vi "PCRE Test.vi"(10 "Values Table":string="{\n \"{test}\": 1\n}", 11 "Expression In":string="({test} == true) OR {b} == false AND {c} == ON") -> (0 "error out":errorcluster, 1 "Reverse Polish Notation Token Stack":cluster{string, string}[](array[cluster]), 2 "Tokens":cluster{string, string}[](array[cluster]), 4 "Total Time":dbl format="%.6fsec", 5 "Result":T1, 6 "Compile Time":dbl format="%.6fsec")   [LabVIEW 2014]
uses:
  src/core/expression/FTW-Expr-BooleanExpressionResult.ctl
  src/core/error/FTW-ERR-ThrowError.vi
  src/core/error/FTW-ERR-CallChain.vi
  src/core/string/FTW-STR-ReplaceWhitespace.vi
  src/core/expression/pcre-8.35/builds/Debug/pcred.dll
  lib/pcre/FTWLib-PCRE32.dll
panel:
  out "Match End":i32
  out "Match Begin":i32
  out "ALL Tokens":cluster{string, string}[](array[cluster])
  out "data string":string
  out "error out 3":errorcluster
  out "LabVIEW PCRE":dbl format="%.4psec"
  out "error out 2":errorcluster
  out "Array":string[](array[string])
  out "Subject":string
  out "Callout Data":T2(array[cluster]) {"callout_id" format="%.0x"; "subject_current_pos" format="%.0x"; "subject_start_match_pos" format="%.0x"; "cap_top" format="%.0x"; "cap_last" format="%.0x"; "patt_pos" format="%.0x"}
  out "Submatches":cluster{i32, i32}[](array[cluster])
  out "PCRE Exec Return":i64
  in  "exec starting offset":i32
  out "Error Offset in Pattern":i64
  out "Error String":string
  out "Pattern":string
  # "({test} == true) OR {b} == false AND {c} == ON"
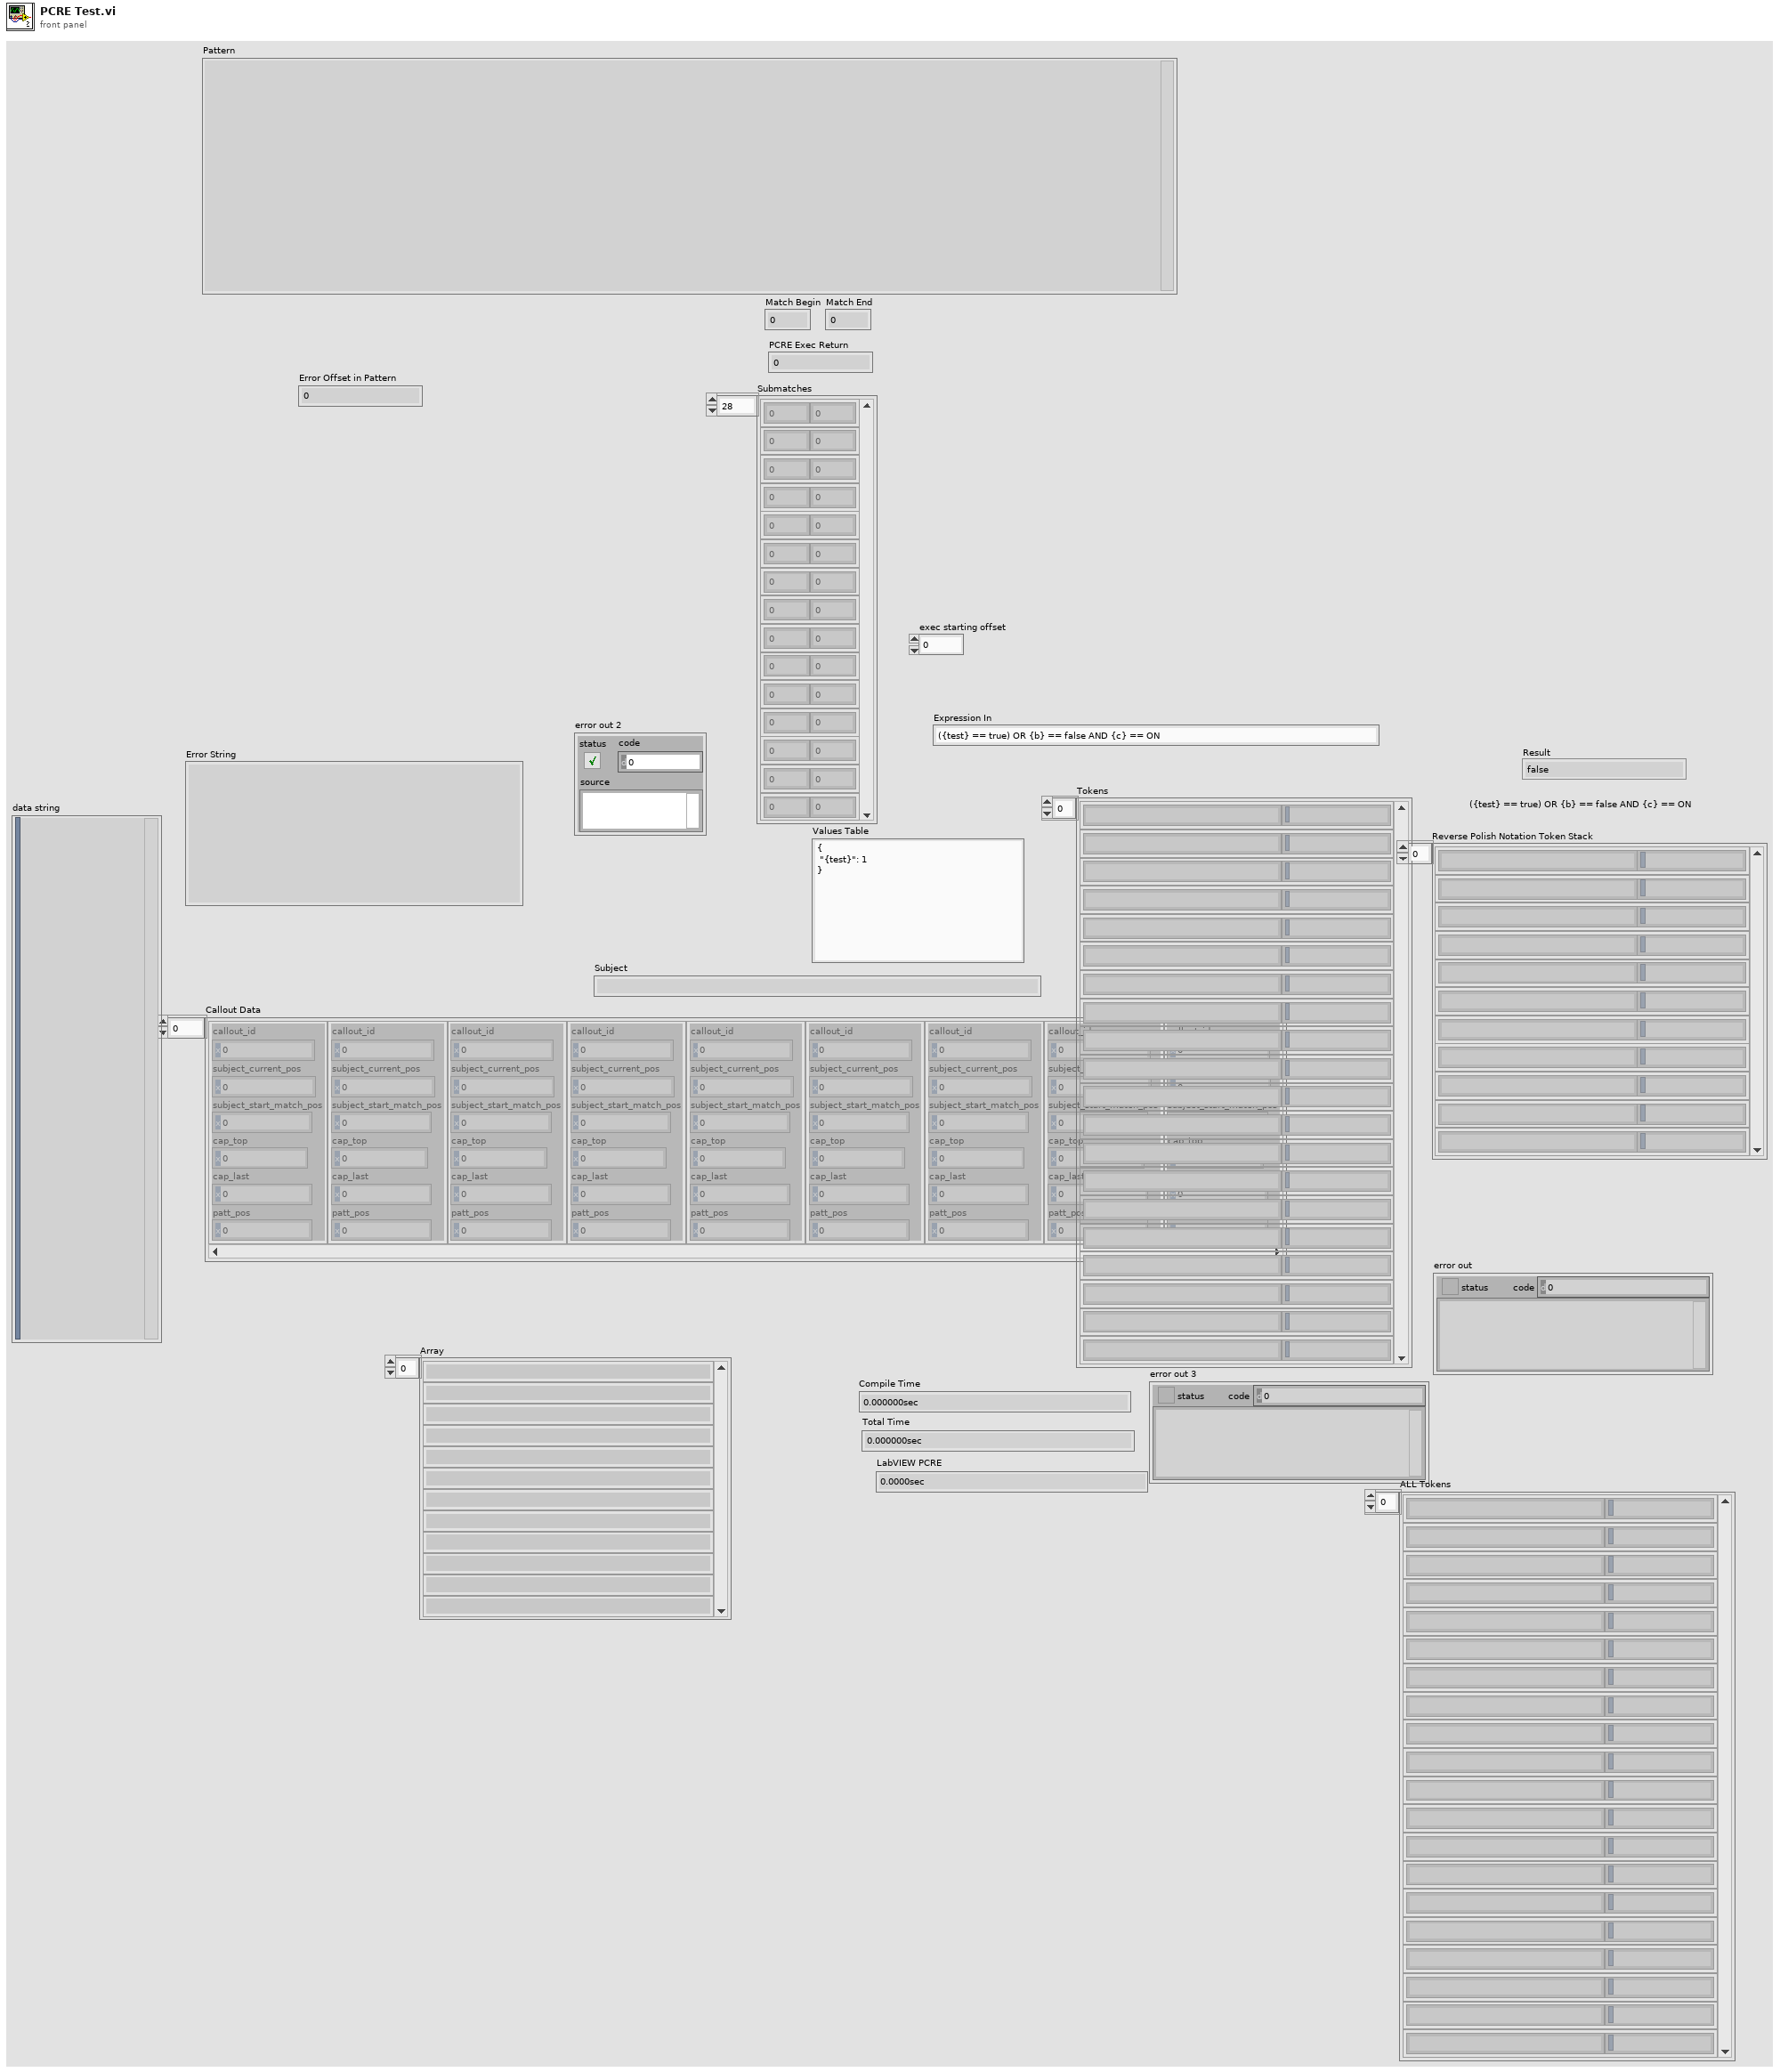
[diagram p1: front panel]
types:
  T1 = typedef "FTW-Expr-BooleanExpressionResult.ctl" = enum16{"false", "true", "inconclusive"}
  T2 = cluster{"callout_id":i32, "subject_current_pos":i32, "subject_start_match_pos":i32, "cap_top":i32, "cap_last":i32, "patt_pos":i32}[]
  T3 = cluster{"op":cluster{"token":string, "value":string}, "Precedence":i32, "Scope Depth":i32}[]
  T4 = cluster{"callout_id":i32, "subject_current_pos":i32, "subject_start_match_pos":i32, "cap_top":i32, "cap_last":i32, "patt_pos":i32}
  T5 = cluster{cluster{"token":string, "value":string}, "Precedence":i32, i32}
  T6 = cluster{"op":cluster{"token":string, "value":string}, "Precedence":i32, "Scope Depth":i32}
  T7 = cluster{cluster{"token":string, "value":string}, "default value 1":i32, "Current Scope Depth":i32}
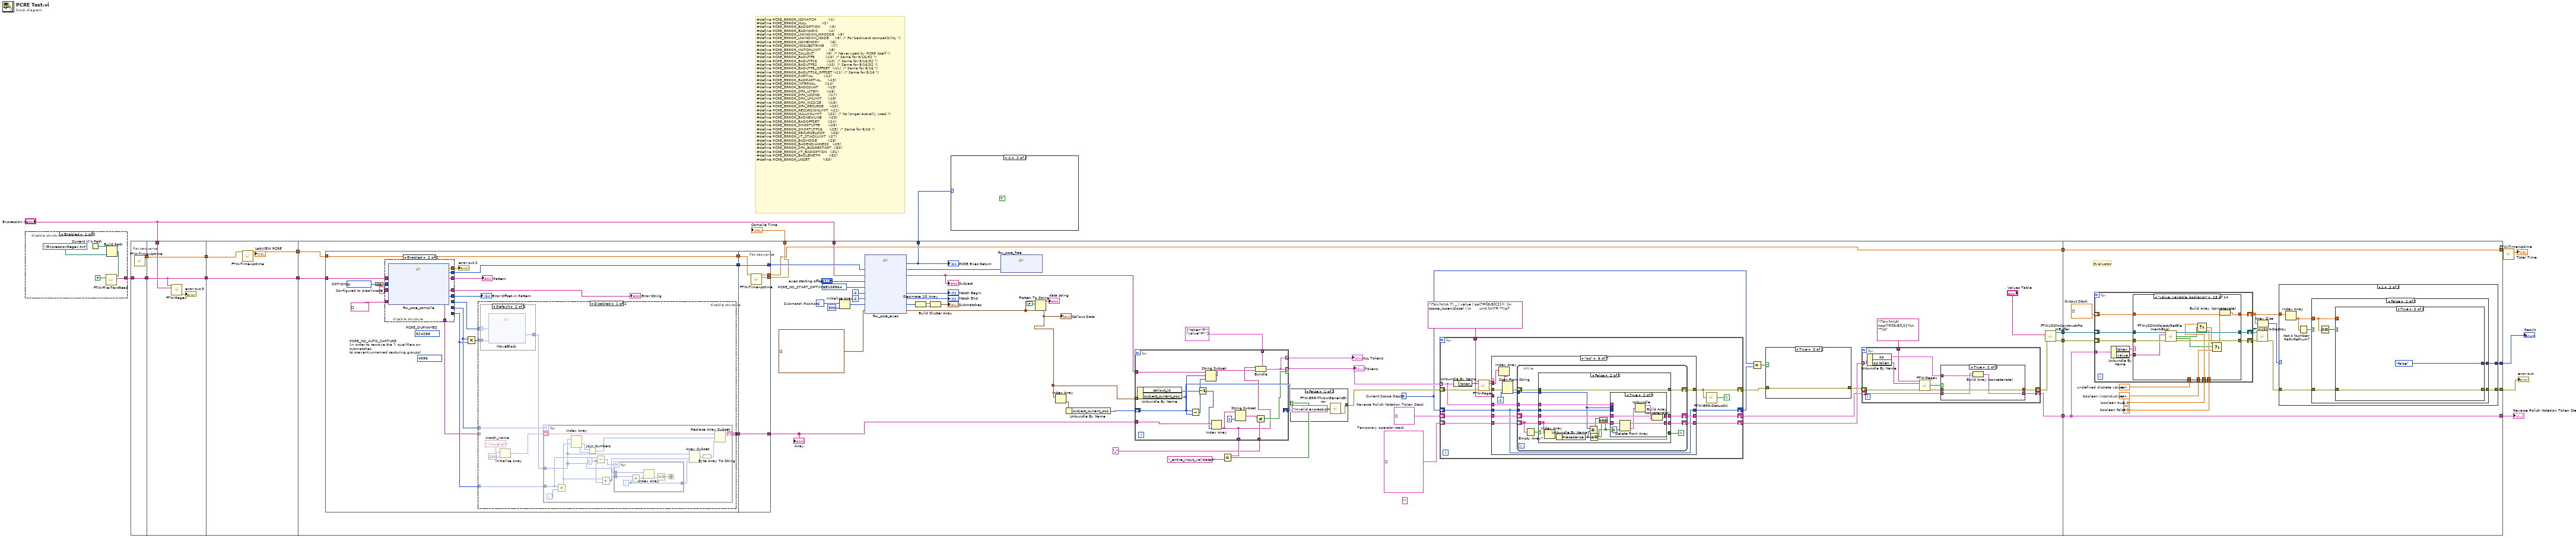
[diagram p0: block diagram]
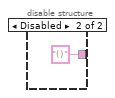
[diagram p3: hidden frame]
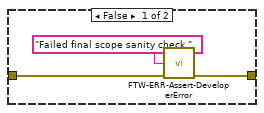
[diagram p4: hidden frame]
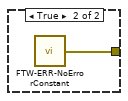
[diagram p5: hidden frame]
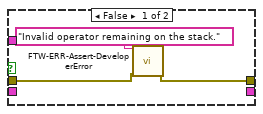
[diagram p6: hidden frame]
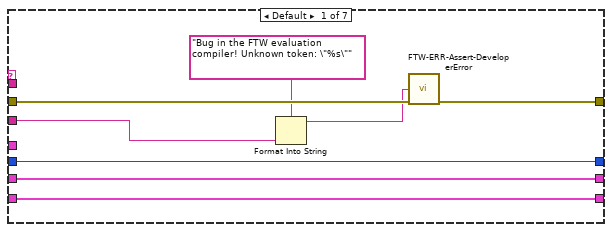
[diagram p7: hidden frame]
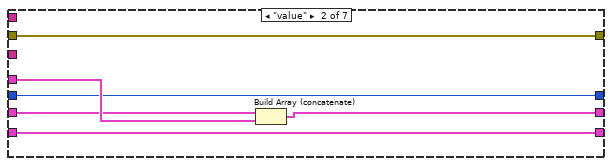
[diagram p8: hidden frame]
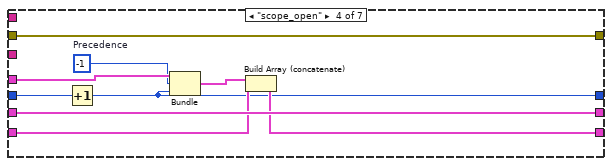
[diagram p10: hidden frame]
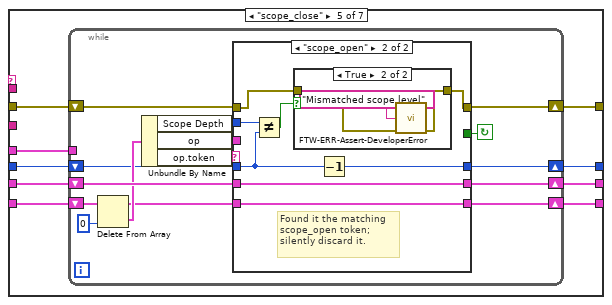
[diagram p11: hidden frame]
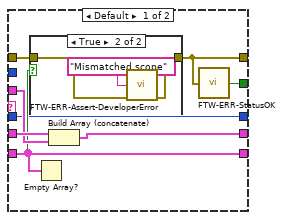
[diagram p12: hidden frame]
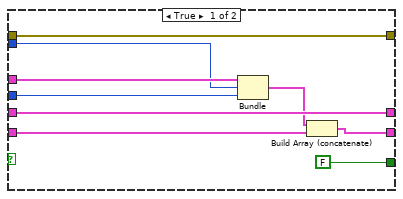
[diagram p15: hidden frame]
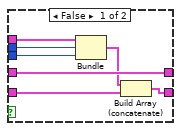
[diagram p16: hidden frame]
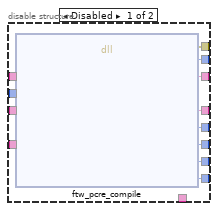
[diagram p20: hidden frame]
diagram:
  # "#define PCRE_ERROR_NOMATCH          (-1)\n#define PCRE_ERROR_NULL             (-2)\n#define PCRE_ERROR_BADOPTION        (-3)\n#define PCRE_ERROR_BADMAGIC         (-4)\n#define PCRE_ERROR_UNKNOWN_OPCODE   (-5)\n#define PCRE_ERROR_UNKNOWN_NODE     (-5)  /* For backward compatibility */\n#define PCRE_ERROR_NOMEMORY         (-6)\n#define PCRE_ERROR_NOSUBSTRING      (-7)\n#define PCRE_ERROR_MATCHLIMIT       (-8)\n#define PCRE_ERROR_CALLOUT          (-9)  /* Never used by PCRE itself */\n#define PCRE_ERROR_BADUTF8         (-10)  /* Same for 8/16/32 */\n#define PCRE_ERROR_BADUTF16        (-10)  /* Same for 8/16/32 */\n#define PCRE_ERROR_BADUTF32        (-10)  /* Same for 8/16/32 */\n#define PCRE_ERROR_BADUTF8_OFFSET  (-11)  /* Same for 8/16 */\n#define PCRE_ERROR_BADUTF16_OFFSET (-11)  /* Same for 8/16 */\n#define PCRE_ERROR_PARTIAL         (-12)\n#define PCRE_ERROR_BADPARTIAL      (-13)\n#define PCRE_ERROR_INTERNAL        (-14)\n#define PCRE_ERROR_BADCOUNT        (-15)\n#define PCRE_ERROR_DFA_UITEM       (-16)\n#define PCRE_ERROR_DFA_UCOND       (-17)\n#define PCRE_ERROR_DFA_UMLIMIT     (-18)\n#define PCRE_ERROR_DFA_WSSIZE      (-19)\n#define PCRE_ERROR_DFA_RECURSE     (-20)\n#define PCRE_ERROR_RECURSIONLIMIT  (-21)\n#define PCRE_ERROR_NULLWSLIMIT     (-22)  /* No longer actually used */\n#define PCRE_ERROR_BADNEWLINE      (-23)\n#define PCRE_ERROR_BADOFFSET       (-24)\n#define PCRE_ERROR_SHORTUTF8       (-25)\n#define PCRE_ERROR_SHORTUTF16      (-25)  /* Same for 8/16 */\n#define PCRE_ERROR_RECURSELOOP     (-26)\n#define PCRE_ERROR_JIT_STACKLIMIT  (-27)\n#define PCRE_ERROR_BADMODE         (-28)\n#define PCRE_ERROR_BADENDIANNESS   (-29)\n#define PCRE_ERROR_DFA_BADRESTART  (-30)\n#define PCRE_ERROR_JIT_BADOPTION   (-31)\n#define PCRE_ERROR_BADLENGTH       (-32)\n#define PCRE_ERROR_UNSET           (-33)"
  n1 = disable-structure shown="Enabled" {
    disable-tunnel: [w21 "()" ("Text")] -> w19
    frame Enabled {
      n2 = Current VI's Path() -> (path=w22:path)
      n3 = Build Path(base path=w22, name or relative path=path "../ExpressionRegex.txt" ("path")) -> (appended path=w20:path)
      n4 = call "FTW-File-TextRead.vi"("Filepath"=w20, "Create if doesn't exist?"=FALSE) -> ("Text"=w21:string)  [unwired: 11 in, 2 out]
    }
    frame Disabled {
    }
  }
  n5 = flat-sequence {
    tunnel: w19 -> [w27]
    tunnel: [w27] -> w6
    tunnel: [w26] -> w2
    tunnel: w6 -> [w31]
    tunnel: [w31] -> w5
    tunnel: "Expression In" -> [w30]
    tunnel: [w29] -> w3
    tunnel: w2 -> [w29]
    tunnel: [w34] -> w16
    tunnel: [w35] -> w14
    tunnel: w5 -> [w34]
    tunnel: w3 -> [w33]
    tunnel: "Expression In" -> [w78]
    tunnel: w16 -> [w83]
    tunnel: w14 -> [w66]
    tunnel: [w61] -> w12
    tunnel: [w57] -> w11
    tunnel: [w67] -> w10
    tunnel: [w62] -> w9
    tunnel: [w60] -> w8
    tunnel: [w36] -> w1
    tunnel: [w379] -> w15
    tunnel: [w378] -> w17
    tunnel: [w370] -> w18
    tunnel: w11 -> [w375]
    tunnel: w10 -> [w378]
    tunnel: w9 -> [w379]
    tunnel: w8 -> [w376]
    tunnel: [w365] -> w7
    frame #0 {
      n6 = call "FTW-Time-Uptime.vi"() -> ("Current Uptime"=w26:dbl)  [unwired: 13 in, 2 out]
    }
    frame #1 {
      n7 = call "FTW-Regex.vi"("Regular Expression"=w31, "Input String"=w30) -> ("error out"=→"error out 3":errorcluster)  [unwired: 9 in, 4 out]
    }
    frame #2 {
      n8 = call "FTW-Time-Uptime.vi"("Previous Uptime"=w33) -> ("Current Uptime"=w35:dbl, "Elapsed Time"=→"LabVIEW PCRE":dbl)  [unwired: 12 in, 1 out]
    }
    frame #3 {
      w39 = -2  # Submatch Position
      (unwired) ""
      w54 = 0  # Current Scope Depth
      w71 = T3 []  # Temporary operator stack
      w72 = cluster{"token":string, "value":string}[] []  # Reverse Polish Notation Token Stack
      w82 = 67108864  # PCRE_NO_START_OPTIMIZE
      n9 = flat-sequence {
        tunnel: w83 -> [w280]
        tunnel: w66 -> [w276]
        tunnel: [w285] -> w65
        tunnel: [w279] -> w64
        tunnel: [w276] -> w63
        tunnel: [w346] -> w80
        tunnel: [w347] -> w90
        tunnel: w65 -> [w347]
        tunnel: w64 -> [w346]
        tunnel: w63 -> [w343]
        tunnel: [w345] -> w62
        tunnel: [w344] -> w61
        frame #0 {
          w273 = ""  # Configured to preallocate
          (unwired) 4096  # PCRE_NO_AUTO_CAPTURE (in order to remove the ?: qualifiers on submatches to prevent unnamed capturing groups)
          (unwired) 524288  # PCRE_DUPNAMES
          w278 = 0  # OPTIONS
          n10 = Compound Arithmetic op=OR(w278) -> (w277:i32)
          n11 = disable-structure shown="Enabled" {
            disable-tunnel: [w332 w342] -> w287
            disable-tunnel: [w331 w341] -> w286
            disable-tunnel: [w330 w340] -> w285
            disable-tunnel: [w329 _] -> w284
            disable-tunnel: [w328 _] -> w282
            disable-tunnel: [w327 _] -> w281
            disable-tunnel: w280 -> [w326 w339]
            disable-tunnel: w277 -> [w325 w338]
            disable-tunnel: [w324 w337] -> w275
            disable-tunnel: [w323 w336] -> w274
            disable-tunnel: w273 -> [w322 w335]
            disable-tunnel: string[] [] ("initialized array") -> [_ w334]
            disable-tunnel: [_ w333] -> w271
            frame Disabled {
              n12 = dll-call lib="C:/Users/Jack/Desktop/app/Sandbox/Expression Lexer/pcre-8.35/builds/Debug/pcred.dll" fn="ftw_pcre_compile"("Pattern"=w326, "Options"=w325, "Error String"=w322) -> (error out=w324:errorcluster, "Compiled Regex"=w330:i64, "Pattern"=w332:string, "Error String"=w323:string, "Error Offset in Pattern"=w331:i64, "Named Capturing Group Table*"=w329:i64, "Named Capturing Group Count"=w328:i32, "Named Capturing Group Length"=w327:i32)  [unwired: 8 in, 1 out]
            }
            frame Enabled {
              n13 = dll-call lib="C:/Users/Jack/repo/ftw-master/ftw/lib/pcre/FTWLib-PCRE32.dll" fn="ftw_pcre_compile"("Pattern"=w339, "Options"=w338, "Error String"=w335, "Named Capturing Group Table"=w334) -> (error out=w337:errorcluster, "Compiled Regex"=w340:i64, "Pattern"=w342:string, "Error String"=w336:string, "Error Offset in Pattern"=w341:i64, "Named Capturing Group Table"=w333:string[])  [unwired: 5 in, 1 out]
            }
          }
          "Pattern" <- w287
          "Error String" <- w274
          "Error Offset in Pattern" <- w286
          "error out 2" <- w275
          n14 = Multiply(x=w282, y=w281) -> (x*y=w283:i32)
          n15 = disable-structure shown="Disabled" {
            disable-tunnel: w284 -> [w296 _]
            disable-tunnel: w283 -> [w295 _]
            disable-tunnel: w282 -> [w294 _]
            disable-tunnel: w281 -> [w293 _]
            disable-tunnel: [w288 w321] -> w279
            disable-tunnel: w271 -> [_ w321]
            frame Disabled {
              w289 = "<invalid>"  # match_name
              n16 = case shown="Default" w296 {
                selector: w296 -> [_ w319]
                tunnel: [_ w320] -> w292
                tunnel: w295 -> [_ w318]
                frame 0 {
                }
                frame Default {
                  n17 = dll-call lib="LabVIEW" fn="MoveBlock"("Source Pointer"=w319, "Buffer Size"=w318) -> ("Destination Buffer"=w320:u8[])  [unwired: 7 in, 2 out]
                }
              }
              n18 = Initialize Array(w289, 256 ("dimension size")) -> (w290:string[])
              n19 = for {
                N: w294 -> [_]
                tunnel: w293 -> [w308]
                tunnel: w292 -> [w304]
                shift-right: [w297] -> w288
                shift-left: w290 -> [w300]
                i -> [w311]
                w306 = 2 ("y")
                n20 = Multiply(x=w308, y=w311) -> (x*y=w305:i32)
                n21 = Index Array(array=w304, index #1=w305) -> (element #1=w310:u8, element #2=w309:u8)  [unwired: 1 in]
                n22 = Join Numbers(hi=w310, lo=w309) -> ((hi.lo)=w299:u16)
                n23 = Subtract(x=w308, y=w306) -> (x-y=w307:i32)
                n24 = Add(x=w305, y=w306) -> (x+y=w301:i32)
                n25 = for {
                  N: w307 -> [_]
                  tunnel: w304 -> [w317]
                  tunnel: w301 -> [w316]
                  tunnel: [w312] -> w302
                  i -> [w312]
                  stop <- w313 stop-if-true
                  n26 = Add(x=w316, y=w312) -> (x+y=w315:i32)
                  n27 = Index Array(array=w317, index=w315) -> (element=w314:u8)
                  n28 = Equal To 0?(x=w314) -> (x = 0?=w313:bool)
                }
                n29 = Array Subset(array=w304, index=w301, length=w302) -> (w303:u8[])
                n30 = Byte Array To String(unsigned byte array=w303) -> (string=w298:string)
                n31 = Replace Array Subset(array=w300, new element=w298, index=w299) -> (w297:string[])
              }
            }
            frame Enabled {
            }
          }
        }
        frame #1 {
          n32 = call "FTW-Time-Uptime.vi"("Previous Uptime"=w343) -> ("Current Uptime"=w345:dbl, "Elapsed Time"=w344:dbl)  [unwired: 12 in, 1 out]
        }
      }
      n33 = Initialize Array(w39, 300 ("dimension size")) -> (w37:i32[])
      n34 = dll-call lib="C:/Users/Jack/repo/ftw-master/ftw/lib/pcre/FTWLib-PCRE32.dll" fn="ftw_pcre_exec"("Compiled Expression"=w90, "Subject String"=w78, "Starting Offset"="exec starting offset", "Options"=w82, "Match Begin"=-2, "Match End"=-2, "Submatch Buffer"=w37, "Callout Buffer"=T2 [] ("*(type *) &x")) -> ("Return Value"=w36:i64, "Compiled Expression"=w49:i64, "Subject String"=w81:string, "Match Begin"=→"Match Begin":i32, "Match End"=→"Match End":i32, "Submatch Buffer"=w89:i32[], "Callout Buffer"=w47:T2)  [unwired: 5 in, 2 out]
      "PCRE Exec Return" <- w36
      "Callout Data" <- w47
      "Subject" <- w81
      n35 = Decimate 1D Array(w89) -> (w88:i32[], w87:i32[])
      n36 = Build Cluster Array(w88, w87) -> (→"Submatches":cluster{i32, i32}[])
      n37 = dll-call lib="C:/Users/Jack/repo/ftw-master/ftw/lib/pcre/FTWLib-PCRE32.dll" fn="ftw_pcre_free"("Compiled Expression"=w49) -> ()  [unwired: 5 in, 2 out]
      n38 = Flatten To String(anything=w47, prepend array or string size? (T)=FALSE) -> (data string=→"data string":string)  [unwired: 2 in, 2 out]
      n39 = Index Array(array=w47) -> (element=w85:T4)  [unwired: 1 in]
      n40 = Unbundle By Name(w85) -> ("subject_current_pos"=w84:i32)
      n41 = for {
        tunnel: w47 -> [w363] mode=indexing
        shift-right: [w360] -> _
        shift-left: w84 -> [w361]
        tunnel: w81 -> [w359]
        tunnel: [w348] -> w75 mode=indexing if=w354
        tunnel: w80 -> [w358]
        tunnel: [w352] -> w77
        tunnel: "_" -> [w356]
        tunnel: cluster{"token":string, "value":string} {"token"="", "value"=""} -> [w353]
        tunnel: [w348] -> w44 mode=indexing
        n42 = Unbundle By Name(w363) -> ("callout_id"=w350:i32, "subject_current_pos"=w360:i32)
        n43 = Subtract(x=w360, y=w361) -> (x-y=w362:i32)
        n44 = Decrement(x=w350) -> (x-1=w349:i32)
        n45 = String Subset(string=w359, offset (0)=w361, length (rest)=w362) -> (substring=w351:string)
        n46 = Index Array(array=w358, index=w349) -> (element=w352:string)
        n47 = String Subset(string=w352, length (rest)=1 ("length (rest)")) -> (substring=w357:string)  [unwired: 1 in]
        n48 = Not Equal?(x=w357, y=w356) -> (x != y?=w354:bool)
        n49 = Bundle(cluster=w353, "token"=w352, "value"=w351) -> (w348:cluster{"token":string, "value":string})
      }
      "Tokens" <- w75
      "ALL Tokens" <- w44
      n50 = Equal?(x=w77, y="_entire_input_validated") -> (x = y?=w56:bool)
      n51 = case shown="False" w56 {
        tunnel: [w96 w98] -> w55
        frame False {
          n52 = call "FTW-ERR-ThrowGenericError.vi"("Error Message"="Invalid expression") -> ("error out"=w96:errorcluster)  [unwired: 14 in]
        }
        frame True {
          n53 = call "FTW-ERR-NoErrorConstant.vi"() -> ("no error"=w98:errorcluster)
        }
      }
      n54 = for {
        tunnel: w75 -> [w127] mode=indexing
        tunnel: "(?six)\n\\A (?: _ | value | op(?=([0-9]{2}))  |\n       scope_(open|close) | \n       unit )\n(?=.*?\\z)" ("Regular Expression") -> [w130]
        shift-right: [w125] -> w68
        shift-left: w72 -> [w126]
        shift-right: [w122] -> w51
        shift-left: w55 -> [w124]
        shift-right: [w120] -> w70
        shift-left: w71 -> [w119]
        shift-right: [w116] -> w53
        shift-left: w54 -> [w117]
        stop <- w121 continue-if-true
        n55 = Unbundle By Name(w127) -> ("token"=w118:string)
        n56 = call "FTW-Regex.vi"("Regular Expression"=w130, "Input String"=w118, "error in"=w124) -> ("Match"=w129:string, "Submatches"=w128:string[], "error out"=w123:errorcluster)  [unwired: 8 in, 2 out]
        n57 = case shown="\"op\"" w129 {
          tunnel: w128 -> [_ _ _ _ _ w209 _]
          tunnel: w127 -> [_ w144 _ w153 w162 w210 _]
          tunnel: w126 -> [w136 w143 w147 w156 w166 w214 w269]
          tunnel: [w136 w142 w147 w156 w164 w215 w269] -> w125
          tunnel: [w137 w141 w148 w157 w161 w212 w270] -> w122
          tunnel: w123 -> [w138 w141 w148 w157 w160 w219 w270]
          tunnel: [w135 w140 w146 w154 w163 w211 w268] -> w120
          tunnel: w119 -> [w135 w140 w146 w155 w165 w216 w268]
          tunnel: w118 -> [w132 _ _ _ _ _ _]
          tunnel: w117 -> [w131 w139 w145 w151 w159 w207 w267]
          tunnel: [w131 w139 w145 w150 w158 w207 w267] -> w116
          frame Default {
            n58 = Format Into String(format string="Bug in the FTW evaluation compiler! Unknown token: \"%s\"" ("Reason this error should never happen"), w132) -> (resulting string=w133:string)  [unwired: 2 in, 1 out]
            n59 = call "FTW-ERR-Assert-DeveloperError.vi"("Reason this error should never happen"=w133, "error in"=w138) -> ("error out"=w137:errorcluster)  [unwired: 13 in]
          }
          frame "value" {
            n60 = Build Array (concatenate)(w143, w144) -> (w142:cluster{"token":string, "value":string}[])
          }
          frame "_" {
            # "As a convention, ignore tokens\nthat begin with this character.\nThey exist in the callout array in\norder to maintain match position."
          }
          frame "scope_open" {
            w149 = -1  # Precedence
            n61 = Increment(x=w151) -> (x+1=w150:i32)
            n62 = Bundle(w153, "Precedence"=w149, w150) -> (w152:T5)  [unwired: 1 in]
            n63 = Build Array (concatenate)(w152, w155) -> (w154:T3)
          }
          frame "scope_close" {
            n64 = while {
              shift-right: [w172] -> w161
              shift-left: w160 -> [w173]
              shift-right: [w181] -> w164
              shift-left: w166 -> [w180]
              shift-right: [w179] -> w163
              shift-left: w165 -> [w178]
              tunnel: w162 -> [_]
              shift-right: [w169] -> w158
              shift-left: w159 -> [w168]
              stop <- w170 continue-if-true
              n65 = Delete From Array(array=w178, index=0) -> (deleted portion=w176:T6, array with subset deleted=w174:T3)  [unwired: 1 in]
              n66 = Unbundle By Name(w176) -> ("Scope Depth"=w167:i32, "op"=w171:cluster{"token":string, "value":string}, "op.token"=w175:string)
              n67 = case shown="\"scope_open\"" w175 {
                tunnel: [w190 w202] -> w181
                tunnel: w180 -> [w189 w202]
                tunnel: [w186 w201] -> w179
                tunnel: w174 -> [w186 w201]
                tunnel: w173 -> [w187 w197]
                tunnel: [w184 w196] -> w172
                tunnel: w171 -> [w188 _]
                tunnel: [w183 _] -> w170
                tunnel: [w182 w200] -> w169
                tunnel: w168 -> [w182 w198]
                tunnel: w167 -> [_ w199]
                frame Default {
                  n68 = Empty Array?(array=w186) -> (empty?=w185:bool)
                  n69 = case shown="True" w185 {
                    tunnel: w187 -> [w191 w194]
                    tunnel: [w191 w192] -> w184
                    frame False {
                    }
                    frame True {
                      n70 = call "FTW-ERR-Assert-DeveloperError.vi"("Reason this error should never happen"="Mismatched scope", "error in"=w194) -> ("error out"=w192:errorcluster)  [unwired: 13 in]
                    }
                  }
                  n71 = Build Array (concatenate)(w189, w188) -> (w190:cluster{"token":string, "value":string}[])
                  n72 = call "FTW-ERR-StatusOK.vi"("error to check"=w184) -> ("Status OK?"=w183:bool)
                }
                frame "scope_open" {
                  # "Found it the matching\nscope_open token;\nsilently discard it."
                  n73 = Not Equal?(x=w199, y=w198) -> (x != y?=w195:bool)
                  n74 = case shown="True" w195 {
                    tunnel: w197 -> [w203 w206]
                    tunnel: [w203 w204] -> w196
                    frame False {
                    }
                    frame True {
                      n75 = call "FTW-ERR-Assert-DeveloperError.vi"("Reason this error should never happen"="Mismatched scope level", "error in"=w206) -> ("error out"=w204:errorcluster)  [unwired: 13 in]
                    }
                  }
                  n76 = Decrement(x=w198) -> (x-1=w200:i32)
                }
              }
            }
          }
          frame "op" {
            n77 = Index Array(array=w209) -> (element=w208:string)  [unwired: 1 in]
            n78 = Scan From String(input string=w208, error in=w219, default 1=-1 ("default value 1")) -> (error out=w213:errorcluster, output 1=w217:i32)  [unwired: 2 in, 2 out]
            n79 = while {
              tunnel: w217 -> [w225]
              shift-right: [w221] -> w212
              shift-left: w213 -> [w220]
              shift-right: [w230] -> w215
              shift-left: w214 -> [w229]
              shift-right: [w228] -> w211
              shift-left: w216 -> [w227]
              tunnel: w210 -> [w226]
              tunnel: w207 -> [w224]
              stop <- w222 continue-if-true
              n80 = Empty Array?(array=w227) -> (empty?=w223:bool)
              n81 = case shown="False" w223 {
                tunnel: [w239 w252] -> w230
                tunnel: w229 -> [w239 w251]
                tunnel: [w238 w250] -> w228
                tunnel: w227 -> [w237 w246]
                tunnel: w226 -> [w236 w249]
                tunnel: w225 -> [w235 w248]
                tunnel: w224 -> [w234 w247]
                tunnel: [FALSE w240] -> w222
                tunnel: [w231 w244] -> w221
                tunnel: w220 -> [w231 w244]
                frame True {
                  n82 = Bundle(w236, "default value 1"=w235, "Current Scope Depth"=w234) -> (w233:T7)  [unwired: 1 in]
                  n83 = Build Array (concatenate)(w233, w237) -> (w238:T3)
                }
                frame False {
                  n84 = Index Array(array=w246) -> (element=w245:T6)  [unwired: 1 in]
                  n85 = Unbundle By Name(w245) -> ("Precedence"=w243:i32)
                  n86 = Greater Or Equal?(x=w248, y=w243) -> (x >= y?=w242:bool)
                  n87 = Greater Or Equal To 0?(x=w243) -> (x >= 0?=w241:bool)
                  n88 = And(x=w242, y=w241) -> (x .and. y?=w240:bool)
                  n89 = case shown="True" w240 {
                    tunnel: [w259 w265] -> w252
                    tunnel: w251 -> [w259 w266]
                    tunnel: [w257 w260] -> w250
                    tunnel: w246 -> [w258 w261]
                    tunnel: w249 -> [w256 _]
                    tunnel: w248 -> [w255 _]
                    tunnel: w247 -> [w253 _]
                    frame False {
                      n90 = Bundle(w256, "default value 1"=w255, "Current Scope Depth"=w253) -> (w254:T7)  [unwired: 1 in]
                      n91 = Build Array (concatenate)(w254, w258) -> (w257:T3)
                    }
                    frame True {
                      n92 = Delete From Array(array=w261, index=0) -> (deleted portion=w263:T6, array with subset deleted=w260:T3)  [unwired: 1 in]
                      n93 = Unbundle(w263) -> ("op"=w262:cluster{"token":string, "value":string})  [unwired: 2 out]
                      n94 = Build Array (concatenate)(w266, w262) -> (w265:cluster{"token":string, "value":string}[])
                    }
                  }
                }
              }
            }
          }
          frame "unit" {
          }
        }
        n95 = call "FTW-ERR-StatusOK.vi"("error to check"=w122) -> ("Status OK?"=w121:bool)
      }
      n96 = Equal?(x=w54, y=w53) -> (x = y?=w52:bool)
      n97 = case shown="True" w52 {
        tunnel: w51 -> [w93 w95]
        tunnel: [w92 w95] -> w50
        frame False {
          n98 = call "FTW-ERR-Assert-DeveloperError.vi"("Reason this error should never happen"="Failed final scope sanity check.", "error in"=w93) -> ("error out"=w92:errorcluster)  [unwired: 13 in]
        }
        frame True {
        }
      }
      n99 = for {
        tunnel: w70 -> [w108] mode=indexing
        shift-right: [w102] -> w58
        shift-left: w50 -> [w107]
        tunnel: "(?six)\n\\A\nop(?=([0-9]{2}))\n.*?\\z" ("Regular Expression") -> [w105]
        shift-right: [w99] -> w67
        shift-left: w68 -> [w100]
        n100 = Unbundle By Name(w108) -> ("op"=w101:cluster{"token":string, "value":string}, "op.token"=w106:string)
        n101 = call "FTW-Regex.vi"("Regular Expression"=w105, "Input String"=w106, "error in"=w107) -> ("Match Found?"=w104:bool, "error out"=w103:errorcluster)  [unwired: 8 in, 3 out]
        n102 = case shown="True" w104 {
          tunnel: w103 -> [w111 w115]
          tunnel: [w109 w115] -> w102
          tunnel: w101 -> [_ w114]
          tunnel: w100 -> [_ w113]
          tunnel: [_ w112] -> w99
          frame False {
            n103 = call "FTW-ERR-Assert-DeveloperError.vi"("Reason this error should never happen"="Invalid operator remaining on the stack.", "error in"=w111) -> ("error out"=w109:errorcluster)  [unwired: 13 in]
          }
          frame True {
            n104 = Build Array (concatenate)(w113, w114) -> (w112:cluster{"token":string, "value":string}[])
          }
        }
      }
      n105 = call "FTW-JSON-Construct-FromBuffer.vi"("JSON String (UTF-8)"="Values Table", "error in"=w58) -> ("JSON Object"=w60:refnum<data-value>, "error out"=w57:errorcluster)  [unwired: 12 in]
      "Array" <- w80
    }
    frame #4 {
      w364 = nan  # undefined discrete value
      w366 = nan  # boolean inconclusive
      w367 = 1.0  # boolean true
      w368 = 0.0  # boolean false
      w377 = dbl[] []  # Output Stack
      # "Evaluator"
      n106 = for {
        tunnel: w378 -> [w423] mode=indexing
        shift-right: [w420] -> w369
        shift-left: w377 -> [w421]
        shift-right: [w418] -> w374
        shift-left: w376 -> [w419]
        shift-right: [w416] -> w373
        shift-left: w375 -> [w417]
        tunnel: w368 -> [w414]
        tunnel: w367 -> [w413]
        tunnel: w366 -> [w412]
        tunnel: w364 -> [w411]
        n107 = Unbundle By Name(w423) -> ("token"=w422:string, "value"=w415:string)
        n108 = case shown="\"value_variable_boolexpr\"" w422 {
          selector: w422 -> [w425 _ _ _ _ _ _ _ _ _ _ _ _ _]
          tunnel: w421 -> [w431 w450 w469 w490 w511 w530 w544 w549 w554 w559 w564 w569 w579 w591]
          tunnel: [w431 w444 w463 w485 w506 w525 w542 w548 w552 w557 w563 w568 w578 w590] -> w420
          tunnel: w419 -> [w430 w443 w462 w484 w505 w524 w541 w547 w551 w556 w562 w567 w583 w595]
          tunnel: [w430 w443 w462 w484 w505 w524 w541 w547 w551 w556 w562 w567 w582 w594] -> w418
          tunnel: w417 -> [w429 w442 w461 w483 w504 w523 w540 w546 w550 w555 w561 w566 w581 w593]
          tunnel: [w428 w442 w461 w483 w504 w523 w540 w546 w550 w555 w561 w566 w580 w592] -> w416
          tunnel: w415 -> [w424 _ _ _ _ _ _ _ _ _ _ _ w577 w589]
          tunnel: w414 -> [_ w434 w453 w477 w498 w517 w533 _ _ _ w560 _ w572 _]
          tunnel: w413 -> [_ w433 w452 w472 w493 w515 w532 w545 _ _ _ _ w573 _]
          tunnel: w412 -> [_ w432 w451 w476 w497 w516 w538 _ _ _ _ w565 w574 _]
          tunnel: w411 -> [_ _ _ _ _ _ _ _ _ _ _ _ _ w587]
          frame Default {
            n109 = Format Into String(format string="Unhandled token '%s' with value '%s'" ("Reason this error should never happen"), w425, w424) -> (resulting string=w427:string)  [unwired: 2 in, 1 out]
            n110 = call "FTW-ERR-Assert-DeveloperError.vi"("Reason this error should never happen"=w427, "error in"=w429) -> ("error out"=w428:errorcluster)  [unwired: 13 in]
          }
          frame "op09_infix_discrete_equal" {
            n111 = Delete From Array(array=w450, index=0) -> (deleted portion=w440:dbl, array with subset deleted=w448:dbl[])  [unwired: 1 in]
            n112 = Delete From Array(array=w448, index=0) -> (deleted portion=w441:dbl, array with subset deleted=w445:dbl[])  [unwired: 1 in]
            n113 = Not A Number/Path/Refnum?(number/path/refnum=w440) -> (NaN/Path/Refnum?=w438:bool)
            n114 = Equal?(x=w441, y=w440) -> (x = y?=w446:bool)
            n115 = Not A Number/Path/Refnum?(number/path/refnum=w441) -> (NaN/Path/Refnum?=w439:bool)
            n116 = Or(x=w439, y=w438) -> (x .or. y?=w437:bool)
            n117 = Select(t=w433, s=w446, f=w434) -> (s? t:f=w436:dbl)
            n118 = Select(t=w432, s=w437, f=w436) -> (s? t:f=w435:dbl)
            n119 = Build Array (concatenate)(w435, w445) -> (w444:dbl[])
          }
          frame "op09_infix_discrete_noteql" {
            n120 = Delete From Array(array=w469, index=0) -> (deleted portion=w459:dbl, array with subset deleted=w467:dbl[])  [unwired: 1 in]
            n121 = Delete From Array(array=w467, index=0) -> (deleted portion=w460:dbl, array with subset deleted=w464:dbl[])  [unwired: 1 in]
            n122 = Not A Number/Path/Refnum?(number/path/refnum=w459) -> (NaN/Path/Refnum?=w457:bool)
            n123 = Not Equal?(x=w460, y=w459) -> (x != y?=w465:bool)
            n124 = Not A Number/Path/Refnum?(number/path/refnum=w460) -> (NaN/Path/Refnum?=w458:bool)
            n125 = Or(x=w458, y=w457) -> (x .or. y?=w456:bool)
            n126 = Select(t=w452, s=w465, f=w453) -> (s? t:f=w455:dbl)
            n127 = Select(t=w451, s=w456, f=w455) -> (s? t:f=w454:dbl)
            n128 = Build Array (concatenate)(w454, w464) -> (w463:dbl[])
          }
          frame "op14_infix_boolexpr_or" {
            n129 = Delete From Array(array=w490, index=0) -> (deleted portion=w473:dbl, array with subset deleted=w488:dbl[])  [unwired: 1 in]
            n130 = Delete From Array(array=w488, index=0) -> (deleted portion=w474:dbl, array with subset deleted=w486:dbl[])  [unwired: 1 in]
            n131 = Equal?(x=w473, y=w472) -> (x = y?=w471:bool)
            n132 = Not A Number/Path/Refnum?(number/path/refnum=w473) -> (NaN/Path/Refnum?=w481:bool)
            n133 = Equal?(x=w474, y=w472) -> (x = y?=w470:bool)
            n134 = Not A Number/Path/Refnum?(number/path/refnum=w474) -> (NaN/Path/Refnum?=w482:bool)
            n135 = Or(x=w470, y=w471) -> (x .or. y?=w475:bool)
            n136 = And(x=w482, y=w481) -> (x .and. y?=w480:bool)
            n137 = Select(t=w472, s=w475, f=w477) -> (s? t:f=w479:dbl)
            n138 = Select(t=w476, s=w480, f=w479) -> (s? t:f=w478:dbl)
            n139 = Build Array (concatenate)(w478, w486) -> (w485:dbl[])
          }
          frame "op13_infix_boolexpr_and" {
            n140 = Delete From Array(array=w511, index=0) -> (deleted portion=w494:dbl, array with subset deleted=w509:dbl[])  [unwired: 1 in]
            n141 = Delete From Array(array=w509, index=0) -> (deleted portion=w495:dbl, array with subset deleted=w507:dbl[])  [unwired: 1 in]
            n142 = Equal?(x=w494, y=w493) -> (x = y?=w492:bool)
            n143 = Not A Number/Path/Refnum?(number/path/refnum=w494) -> (NaN/Path/Refnum?=w502:bool)
            n144 = Equal?(x=w495, y=w493) -> (x = y?=w491:bool)
            n145 = Not A Number/Path/Refnum?(number/path/refnum=w495) -> (NaN/Path/Refnum?=w503:bool)
            n146 = And(x=w491, y=w492) -> (x .and. y?=w496:bool)
            n147 = Or(x=w503, y=w502) -> (x .or. y?=w501:bool)
            n148 = Select(t=w493, s=w496, f=w498) -> (s? t:f=w500:dbl)
            n149 = Select(t=w497, s=w501, f=w500) -> (s? t:f=w499:dbl)
            n150 = Build Array (concatenate)(w499, w507) -> (w506:dbl[])
          }
          frame "op09_infix_boolexpr_xor" {
            n151 = Delete From Array(array=w530, index=0) -> (deleted portion=w513:dbl, array with subset deleted=w528:dbl[])  [unwired: 1 in]
            n152 = Not A Number/Path/Refnum?(number/path/refnum=w513) -> (NaN/Path/Refnum?=w521:bool)
            n153 = Delete From Array(array=w528, index=0) -> (deleted portion=w512:dbl, array with subset deleted=w526:dbl[])  [unwired: 1 in]
            n154 = Not A Number/Path/Refnum?(number/path/refnum=w512) -> (NaN/Path/Refnum?=w522:bool)
            n155 = Not Equal?(x=w512, y=w513) -> (x != y?=w514:bool)
            n156 = Or(x=w522, y=w521) -> (x .or. y?=w520:bool)
            n157 = Select(t=w515, s=w514, f=w517) -> (s? t:f=w519:dbl)
            n158 = Select(t=w516, s=w520, f=w519) -> (s? t:f=w518:dbl)
            n159 = Build Array (concatenate)(w518, w526) -> (w525:dbl[])
          }
          frame "op03_prefix_boolexpr_not" {
            n160 = Delete From Array(array=w544, index=0) -> (deleted portion=w535:dbl, array with subset deleted=w537:dbl[])  [unwired: 1 in]
            n161 = Not A Number/Path/Refnum?(number/path/refnum=w535) -> (NaN/Path/Refnum?=w536:bool)
            n162 = Equal?(x=w535, y=w532) -> (x = y?=w534:bool)
            n163 = Select(t=w533, s=w534, f=w532) -> (s? t:f=w531:dbl)
            n164 = Select(t=w538, s=w536, f=w531) -> (s? t:f=w539:dbl)
            n165 = Build Array (concatenate)(w539, w537) -> (w542:dbl[])
          }
          frame "value_const_boolexpr_true" {
            n166 = Build Array (concatenate)(w545, w549) -> (w548:dbl[])
          }
          frame "value_const_discrete1" {
            w553 = 1.0  # discrete 1
            n167 = Build Array (concatenate)(w553, w554) -> (w552:dbl[])
          }
          frame "value_const_discrete0" {
            w558 = 0.0  # discrete 0
            n168 = Build Array (concatenate)(w558, w559) -> (w557:dbl[])
          }
          frame "value_const_boolexpr_false" {
            n169 = Build Array (concatenate)(w560, w564) -> (w563:dbl[])
          }
          frame "value_const_undefined" {
            n170 = Build Array (concatenate)(w565, w569) -> (w568:dbl[])
          }
          frame "value_variable_boolexpr" {
            n171 = call "FTW-JSON-Object-GetElement-Bool.vi"("JSON Object"=w583, "Key"=w577, "error in"=w581) -> ("JSON Object out"=w582:refnum<data-value>, "Value"=w570:bool, "Found?"=w571:bool, "error out"=w580:errorcluster)  [unwired: 9 in]
            n172 = Select(t=w573, s=w570, f=w572) -> (s? t:f=w576:dbl)
            n173 = Select(t=w576, s=w571, f=w574) -> (s? t:f=w575:dbl)
            n174 = Build Array (concatenate)(w575, w579) -> (w578:dbl[])
          }
          frame "value_variable_discrete" {
            n175 = call "FTW-JSON-Object-GetElement-Integer.vi"("JSON Object"=w595, "Key"=w589, "error in"=w593) -> ("JSON Object out"=w594:refnum<data-value>, "Value"=w585:i32, "Found?"=w584:bool, "error out"=w592:errorcluster)  [unwired: 9 in]
            n176 = To Double Precision Float(number=w585) -> (double precision float=w586:dbl)
            n177 = Select(t=w586, s=w584, f=w587) -> (s? t:f=w588:dbl)
            n178 = Build Array (concatenate)(w588, w591) -> (w590:dbl[])
          }
        }
      }
      n179 = call "FTW-JSON-Destroy.vi"("JSON Object"=w374, "error in"=w373) -> ("error out"=w371:errorcluster)  [unwired: 13 in]
      n180 = Array Size(array=w369) -> (size(s)=w372:i32)
      n181 = case shown="1" w372 {
        tunnel: w371 -> [w383 w387]
        tunnel: [w382 w388] -> w370
        tunnel: w369 -> [_ w389]
        tunnel: [FTW-Expr-BooleanExpressionResult."inconclusive" ("Result") w385] -> w365
        frame Default {
          n182 = call "FTW-ERR-Assert-DeveloperError.vi"("Reason this error should never happen"="Evaluation stack has items remaining!", "error in"=w383) -> ("error out"=w382:errorcluster)  [unwired: 13 in]
        }
        frame 1 {
          n183 = Index Array(array=w389) -> (element=w384:dbl)  [unwired: 1 in]
          n184 = Not A Number/Path/Refnum?(number/path/refnum=w384) -> (NaN/Path/Refnum?=w386:bool)
          n185 = case shown="False" w386 {
            tunnel: [w394 w409] -> w388
            tunnel: w387 -> [w393 w409]
            tunnel: [w391 FTW-Expr-BooleanExpressionResult."inconclusive" ("Result")] -> w385
            tunnel: w384 -> [w390 _]
            frame False {
              n186 = Equal To 0?(x=w390) -> (x = 0?=w392:bool)
              n187 = case shown="True" w392 {
                tunnel: [w399 w408] -> w394
                tunnel: w393 -> [w400 w408]
                tunnel: [w395 FTW-Expr-BooleanExpressionResult."false" ("Result")] -> w391
                tunnel: w390 -> [w398 _]
                frame False {
                  n188 = Equal?(x=w398, y=1.0) -> (x = y?=w396:bool)
                  n189 = case shown="True" w396 {
                    tunnel: w400 -> [w403 w405]
                    tunnel: [w402 w405] -> w399
                    tunnel: [FTW-Expr-BooleanExpressionResult."inconclusive" ("Result") FTW-Expr-BooleanExpressionResult."true" ("Result")] -> w395
                    frame False {
                      n190 = call "FTW-ERR-Assert-DeveloperError.vi"("Reason this error should never happen"="Boolean expression evaluated to non-Boolean result!", "error in"=w403) -> ("error out"=w402:errorcluster)  [unwired: 13 in]
                    }
                    frame True {
                    }
                  }
                }
                frame True {
                }
              }
            }
            frame True {
            }
          }
        }
      }
    }
  }
  n191 = case shown="-1" w1 {
    frame Default {
    }
    frame -1 {
      (unwired) TRUE
    }
  }
  n192 = call "FTW-Time-Uptime.vi"("Previous Uptime"=w15) -> ("Elapsed Time"=→"Total Time":dbl)  [unwired: 12 in, 2 out]
  "error out" <- w18
  "Reverse Polish Notation Token Stack" <- w17
  "Compile Time" <- w12
  "Result" <- w7
